vi "10.3-actual.vi"() -> ()   [LabVIEW 2012]
panel:
  out "Desired DAC ouput":dbl
  out "Actual DAC output":dbl
  out "DAC Output":cluster{"Y":dbl[], "Y":dbl[]}[](graph)
  out "DAC Deviation":cluster{"Y":dbl[], "Y":dbl[]}[](graph)
  out "Bit Pattern":i32 format="%b"
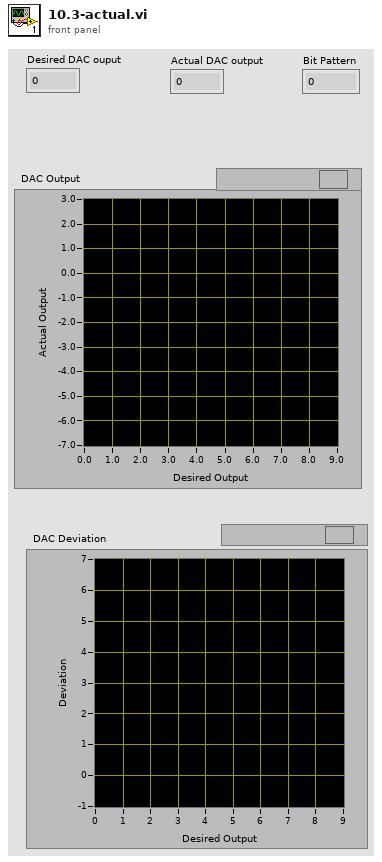
[diagram p1: front panel]
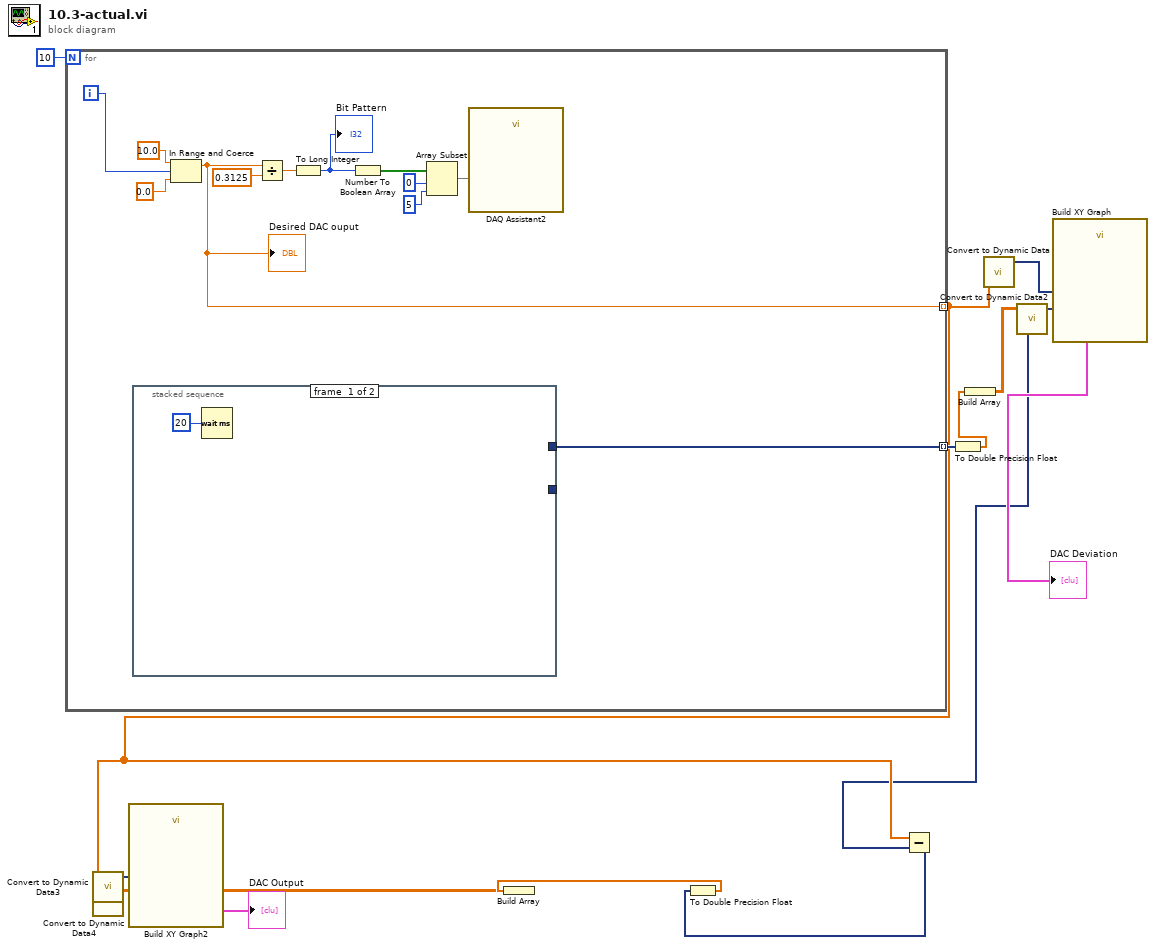
[diagram p0: block diagram]
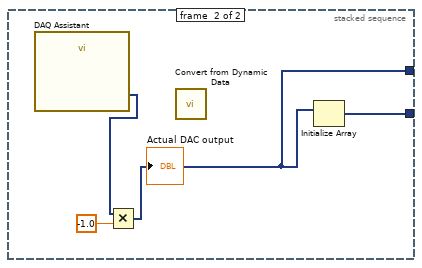
[diagram p2: hidden frame]
diagram:
  n1 = for {
    N: 10 -> [_]
    tunnel: [w17] -> w6 mode=indexing
    tunnel: [w16] -> w11 mode=indexing
    i -> [w15]
    n2 = stacked-sequence {
      tunnel: [_ w31] -> _
      tunnel: [_ w29] -> w16
      frame #0 {
        n3 = Wait (ms)(milliseconds to wait=20) -> ()  [unwired: 1 out]
      }
      frame #1 {
        n4 = call "DAQ Assistant"() -> ("data"=w28:dynamicdata)  [unwired: 17 in, 2 out]
        n5 = Multiply(x=w28, y=-1.0) -> (x*y=w29:dynamicdata)
        "Actual DAC output" <- w29
        n6 = call "Convert from Dynamic Data"() -> ()  [unwired: 4 in, 1 out]
        n7 = Initialize Array(w29) -> (w31:dynamicdata[])  [unwired: 1 in]
      }
    }
    n8 = In Range and Coerce(upper limit=10.0, x=w15, lower limit=0.0) -> (coerced(x)=w17:dbl)  [unwired: 1 out]
    "Desired DAC ouput" <- w17
    n9 = Divide(x=w17, y=0.3125) -> (x/y=w23:dbl)
    n10 = To Long Integer(number=w23) -> (32bit integer=w22:i32)
    "Bit Pattern" <- w22
    n11 = Number To Boolean Array(number=w22) -> (Boolean array=w21:bool[])
    n12 = Array Subset(array=w21, index=0, length=5) -> (w18:bool[])
    n13 = call "DAQ Assistant2"("data"=w18) -> ()  [unwired: 17 in, 2 out]
  }
  n14 = call "Convert to Dynamic Data3"("Array"=w6) -> ("Dynamic Data Type"=w8:dynamicdata)  [unwired: 3 in]
  n15 = To Double Precision Float(number=w11) -> (double precision float=w10:dbl[])
  n16 = Build Array(w10) -> (w7:dbl[][])
  n17 = call "Convert to Dynamic Data"("Array"=w6) -> ("Dynamic Data Type"=w13:dynamicdata)  [unwired: 3 in]
  n18 = call "Convert to Dynamic Data2"("2D Array"=w7) -> ("Dynamic Data Type"=w5:dynamicdata)  [unwired: 3 in]
  n19 = Subtract(x=w6, y=w5) -> (x-y=w4:dynamicdata[])
  n20 = To Double Precision Float(number=w4) -> (double precision float=w3:dbl[])
  n21 = Build Array(w3) -> (w2:dbl[][])
  n22 = call "Convert to Dynamic Data4"("2D Array"=w2) -> ("Dynamic Data Type"=w1:dynamicdata)  [unwired: 3 in]
  n23 = call "Build XY Graph2"("Y Input"=w1, "X Input"=w8) -> ("XY Graph"=→"DAC Output":cluster{"Y":dbl[], "Y":dbl[]}[])  [unwired: 3 in, 6 out]
  n24 = call "Build XY Graph"("Y Input"=w5, "X Input"=w13) -> ("XY Graph"=→"DAC Deviation":cluster{"Y":dbl[], "Y":dbl[]}[])  [unwired: 3 in, 6 out]
